vi "skalowanie wykresu - test.vi"() -> ()   [LabVIEW 2013]
panel:
  out "Waveform Graph 2":waveform(dbl)(graph)
  in  "Zakres wysw":dbl
  in  "stop":bool
  out "Waveform Graph":waveform(dbl)(graph)
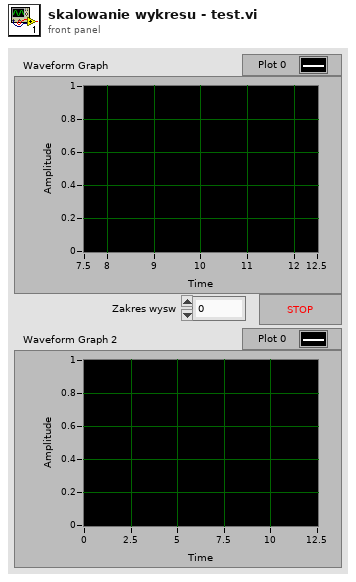
[diagram p1: front panel]
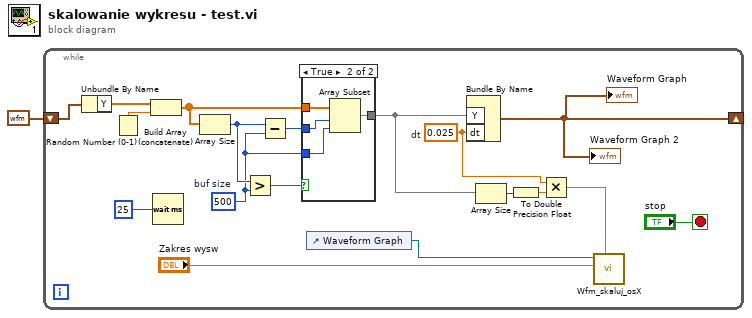
[diagram p0: block diagram]
diagram:
  n1 = while {
    shift-right: [w7] -> _
    shift-left: waveform(dbl) {"t0"=timestamp(0 s since 1904-01-01), "dt"=1.0, "Y"=[]} -> [w9]
    stop <- "stop" stop-if-true
    w5 = 0.025  # dt
    w11 = 500  # buf size
    n2 = Unbundle By Name(w9) -> ("Y"=w8:dbl[])
    n3 = Random Number (0-1)() -> (number: 0 to 1=w18:dbl)
    n4 = Build Array (concatenate)(w8, w18) -> (w16:dbl[])
    n5 = Wait (ms)(milliseconds to wait=u32 25) -> ()  [unwired: 1 out]
    n6 = Array Size(array=w16) -> (size(s)=w12:i32)
    n7 = Greater?(x=w12, y=w11) -> (0:w15:bool)
    n8 = Subtract(x=w12, y=w11) -> (x-y=w14:i32)
    n9 = case shown="True" w15 {
      tunnel: [w20 w24] -> w6
      tunnel: w16 -> [w20 w23]
      tunnel: w14 -> [_ w22]
      tunnel: w11 -> [_ w21]
      frame False {
      }
      frame True {
        n10 = Array Subset(array=w23, index=w22, length=w21) -> (w24:dbl[])
      }
    }
    n11 = control-ref of="Waveform Graph"() -> (w10:refnum<vi>)
    n12 = Bundle By Name("Y"=w6, "dt"=w5) -> (w7:waveform(dbl))  [unwired: 1 in]
    "Waveform Graph" <- w7
    "Waveform Graph 2" <- w7
    n13 = Array Size(array=w6) -> (size(s)=w2:i32)
    n14 = To Double Precision Float(number=w2) -> (double precision float=w3:dbl)
    n15 = Multiply(x=w5, y=w3) -> (x*y=w4:dbl)
    n16 = call "Wfm_skaluj_osX.vi"("size(s)"=w4, "Zakres wysw"="Zakres wysw", "Waveform in"=w10) -> ()  [unwired: 8 in, 1 out]
  }
